vi "acq_data.vi"(8 "error in":errorcluster, 11 "MainFGV_data in":T1={"TestDir"=path "", "TestName"="", "task"="", "data_file"=refnum, "AcqQueue"=refnum, "StartTime"=timestamp(0 s since 1904-01-01), "config_channels"=[], "DAQmx Device"="", "Advanced"={"rate"=0.0, "duration"=0.0, "thr"=0.0, "preTrigger"=0.0, "cutoff"=0.0, "Filtro"=enum."Desativado", "highPass"=0.0, "lowPass"=0.0, "updateTime"=0.0}, "running"=FALSE, "hammerIndex"=0, "session"="localhost"} {"Advanced"."updateTime" format="%#_g ms"; "Advanced"."lowPass" format="%#_g Hz"; "Advanced"."highPass" format="%#_g Hz"; "Advanced"."cutoff" format="%#_g dB"; "Advanced"."preTrigger" format="%#_g ms"; "Advanced"."thr" format="%#_g N"; "Advanced"."duration" format="%#_g s"; "Advanced"."rate" min=1652.0 max=51200.0 format="%#_g Hz"}) -> (0 "error out":errorcluster)   [LabVIEW 2018]
uses:
  MainFGV_data.ctl
  Settings/config_board.ctl
  Settings/Advanced/AdvancedConfig.ctl
  <vilib>/DAQmx/read.llb/DAQmx Read (Analog 2D DBL NChan NSamp).vi
  <vilib>/DAQmx/miscellaneous.llb/DAQmx Fill In Error Info.vi
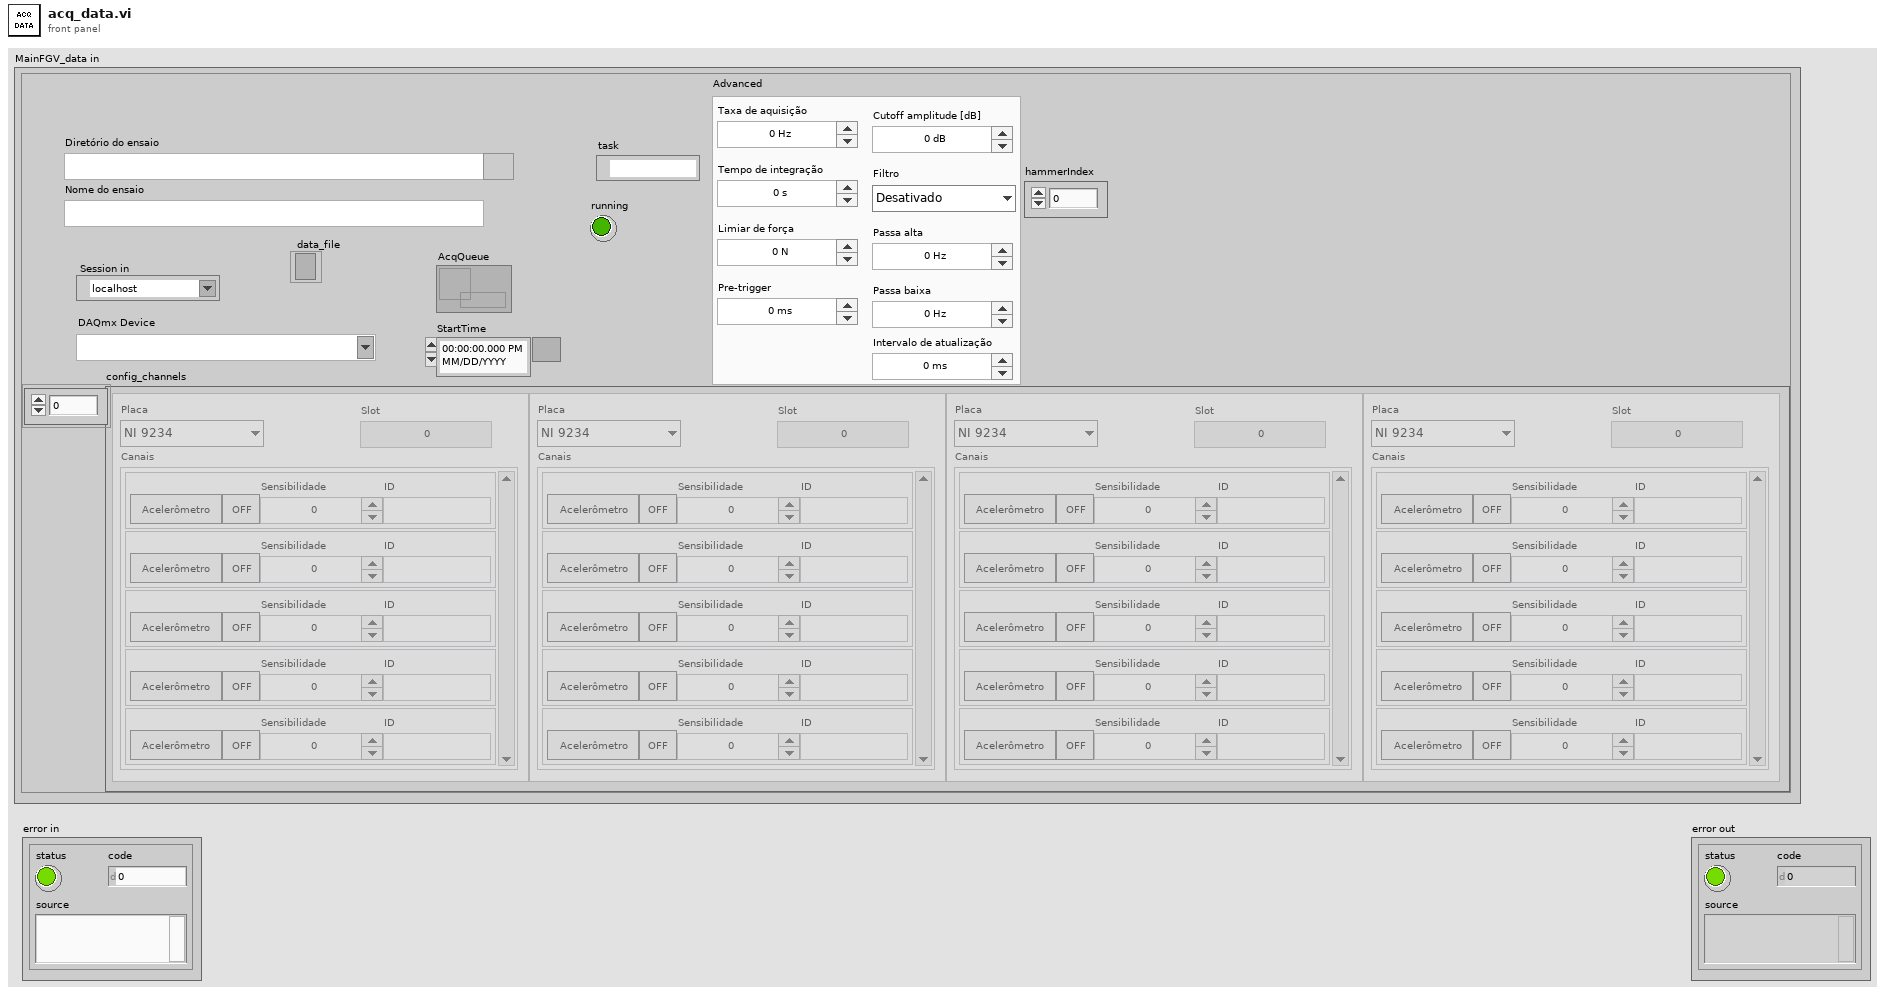
[diagram p1: front panel]
types:
  T1 = typedef "MainFGV_data.ctl" = cluster{"TestDir":path, "TestName":string, "task":refnum<k21>, "data_file":refnum<file>, "AcqQueue":refnum<queue>, "StartTime":timestamp, "config_channels":T2[], "DAQmx Device":tag, "Advanced":T3, "running":bool, "hammerIndex":i32, "session":refnum<k21>}
  T2 = typedef "config_board.ctl" = cluster{"board":enum16{"NI 9234", "NI 9205", "Não aplicável"}, "channels":cluster{"type":bool, "active":bool, "sens":dbl, "ID":string}[], "Slot":i32}
  T3 = typedef "AdvancedConfig.ctl" = cluster{"rate":dbl, "duration":dbl, "thr":dbl, "preTrigger":dbl, "cutoff":dbl, "Filtro":enum16{"Desativado", "Passa banda", "Passa alta", "Passa baixa"}, "highPass":dbl, "lowPass":dbl, "updateTime":dbl}
  T4 = cluster{"type":bool, "active":bool, "sens":dbl, "ID":string}[]
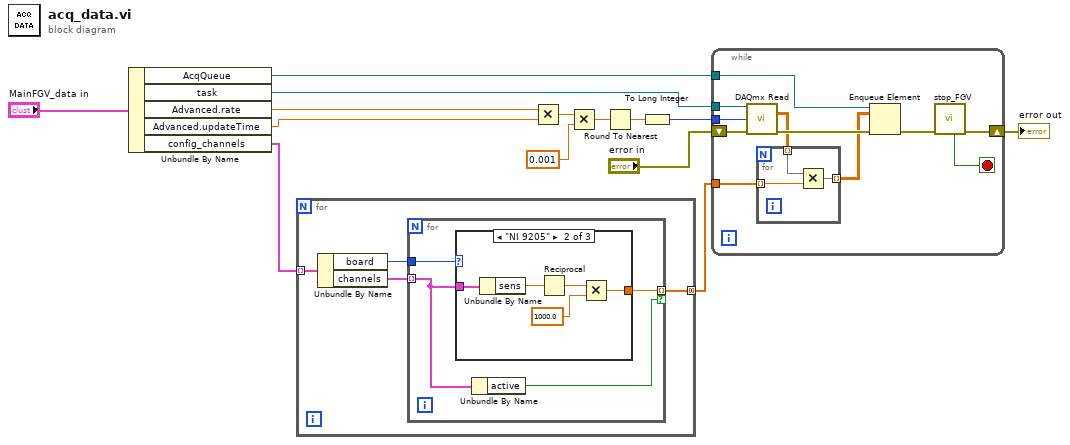
[diagram p0: block diagram]
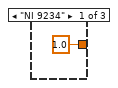
[diagram p2: hidden frame]
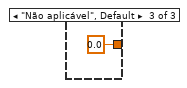
[diagram p3: hidden frame]
diagram:
  n1 = Unbundle By Name("MainFGV_data in") -> ("AcqQueue"=w6:refnum<queue>, "task"=w5:refnum<k21>, "Advanced.rate"=w10:dbl, "Advanced.updateTime"=w9:dbl, "config_channels"=w2:T2[])
  n2 = for {
    tunnel: w2 -> [w18] mode=indexing
    tunnel: [w15] -> w1 mode=concatenating
    n3 = Unbundle By Name(w18) -> ("board"=w17:enum16{"NI 9234", "NI 9205", "Não aplicável"}, "channels"=w16:T4)
    n4 = for {
      tunnel: w17 -> [w22]
      tunnel: w16 -> [w20] mode=indexing
      tunnel: [w21] -> w15 mode=indexing if=w19
      n5 = case shown="\"NI 9205\"" w22 {
        tunnel: w20 -> [_ w28 _]
        tunnel: [1.0 w24 0.0] -> w21
        frame "NI 9234" {
        }
        frame "NI 9205" {
          n6 = Unbundle By Name(w28) -> ("sens"=w27:dbl)
          n7 = Reciprocal(x=w27) -> (1/x=w26:dbl)
          n8 = Multiply(x=w26, y=1000.0) -> (x*y=w24:dbl)
        }
        frame "Não aplicável", Default {
        }
      }
      n9 = Unbundle By Name(w20) -> ("active"=w19:bool)
    }
  }
  n10 = Multiply(x=w10, y=w9) -> (x*y=w8:dbl)
  n11 = Multiply(x=w8, y=0.001) -> (x*y=w12:dbl)
  n12 = Round To Nearest(number=w12) -> (nearest integer value=w7:dbl)
  n13 = To Long Integer(number=w7) -> (32bit integer=w11:i32)
  n14 = while {
    tunnel: w11 -> [w39]
    tunnel: w6 -> [w38]
    tunnel: w5 -> [w37]
    shift-right: [w34] -> w14
    shift-left: "error in" -> [w36]
    tunnel: w1 -> [w32]
    stop <- w33 stop-if-true
    n15 = call-poly <vilib>:"DAQmx Read.vi"("task/channels in"=w37, "number of samples per channel"=w39, "error in"=w36) -> ("data"=w31:dbl[][], "error out"=w40:errorcluster)  [unwired: 10 in, 1 out]
    n16 = for {
      tunnel: w31 -> [w43] mode=indexing
      tunnel: w32 -> [w42] mode=indexing
      tunnel: [w41] -> w30 mode=indexing
      n17 = Multiply(x=w43, y=w42) -> (x*y=w41:dbl[])
    }
    n18 = Enqueue Element(queue=w38, element=w30, error in (no error)=w40) -> (error out=w35:errorcluster)  [unwired: 1 in, 2 out]
    n19 = call "stop_FGV.vi"("error in (no error)"=w35) -> ("error out"=w34:errorcluster, "parar?"=w33:bool)  [unwired: 9 in]
  }
  "error out" <- w14
